vi "Kikusui PLZ-Configure Operation.vi"(8 "error in":errorcluster, 10 "Operation Mode (0:Constant Current)":u16(ring) items=["Constant Current(CC)", "Constant Voltage(CV)", "Constant Power(CP)", "Constant Resistance(CR)", "Constant Current & Voltage(CCCV)", "Constant Resistance & Voltage(CRCV)"], 11 "Kikusui PLZ Setting In":T1={"VISA Resource Name"="", "Baud Rate"=19200, "Stop Bits"=20, "Wait For Read(ms)"=0} {"Stop Bits" items=["1.0"=10, "2.0"=20]; "Baud Rate" items=["2400"=2400, "4800"=4800, "9600"=9600, "19200"=19200]}) -> (0 "error out":errorcluster, 3 "Kikusui PLZ Setting Out":T1={"VISA Resource Name"="", "Baud Rate"=19200, "Stop Bits"=20, "Wait For Read(ms)"=0} {"Stop Bits" items=["1.0"=10, "2.0"=20]; "Baud Rate" items=["2400"=2400, "4800"=4800, "9600"=9600, "19200"=19200]})   [LabVIEW 2018]
doc: "Configures the operation mode of the instrument."
uses:
  Data Def/Kikusui PLZ-Setting.ctl
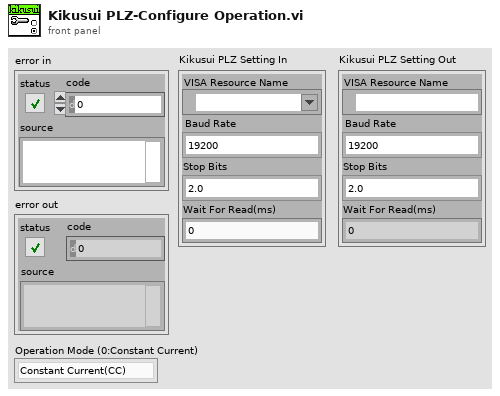
[diagram p1: front panel]
types:
  T1 = typedef "Kikusui PLZ-Setting.ctl" = cluster{"VISA Resource Name":refnum<visa-resource-name>, "Baud Rate":u32, "Stop Bits":u16, "Wait For Read(ms)":u32}
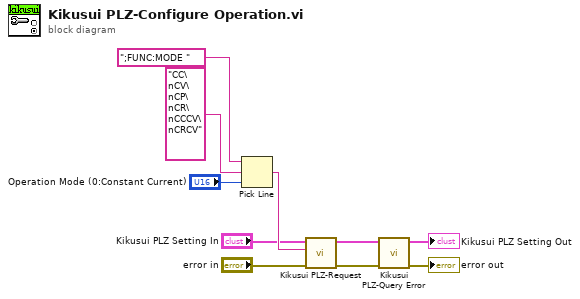
[diagram p0: block diagram]
diagram:
  n1 = Pick Line(string ("")=";FUNC:MODE ", multi-line string="CC\nCV\nCP\nCR\nCCCV\nCRCV", line index="Operation Mode (0:Constant Current)") -> (output string=w6:string)
  n2 = call "Kikusui PLZ-Request.vi"("error in"="error in", "Command"=w6, "Kikusui PLZ Setting In"="Kikusui PLZ Setting In") -> ("error out"=w5:errorcluster, "Kikusui PLZ Setting Out"=w4:T1)  [unwired: 6 in, 1 out]
  n3 = call "Kikusui PLZ-Query Error.vi"("error in"=w5, "Kikusui PLZ Setting In"=w4) -> ("error out"=→"error out":errorcluster, "Kikusui PLZ Setting Out"=→"Kikusui PLZ Setting Out":T1)  [unwired: 8 in]
